vi "Read Digital Outputs Status.vi"(8 "error in (no error)":errorcluster, 11 "PXI6521 in":refnum<class "PXI6521.lvclass">) -> (0 "error out":errorcluster, 2 "Digital Outputs Status":bool[](array[boolean]), 3 "PXI6521 out":refnum<class "PXI6521.lvclass">)   [LabVIEW 2018, in "PXI6521.lvlib" / "PXI6521.lvclass"]
doc: "This VI reads the state of the Digital Outputs. The state is atores in the applicable class property."
uses:
  PXI6521.lvclass
  Custom Controls/DAQmx Lines Scope.ctl
  Custom Controls/DAQmx Digital Scope.ctl
  PXI6521.lvclass/PXI6521.ctl
  <vilib>/DAQmx/read.llb/DAQmx Read (Digital 1D Bool 1Chan 1Samp).vi
  <vilib>/DAQmx/create/channels.llb/DAQmx Create Channel (DO-Digital Output).vi
  <vilib>/DAQmx/miscellaneous.llb/DAQmx Fill In Error Info.vi
  PPLs/DigitalIO/Parent/DigitalIO.lvlibp/DigitalIO.lvclass
  C:/Projects/LabVIEW/PPLs/DigitalIO/Parent/DigitalIO.lvlibp/DigitalIO.lvclass
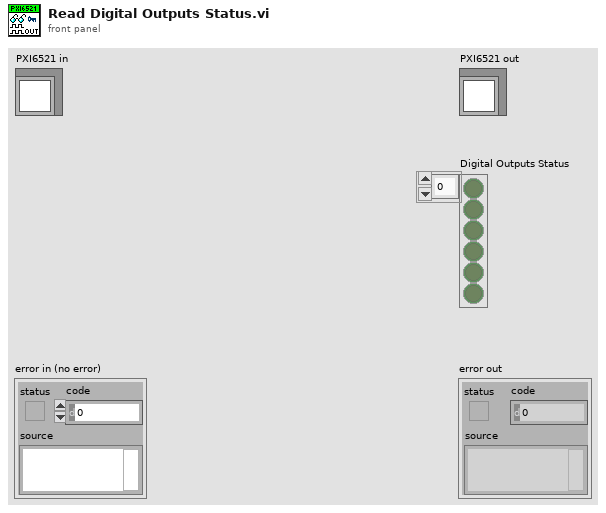
[diagram p1: front panel]
types:
  T1 = typedef "PXI6521.lvlib/PXI6521.lvclass/DAQmx Digital Scope.ctl" = enum16{"Input", "Output"}
  T2 = typedef "PXI6521.lvlib/PXI6521.lvclass/DAQmx Lines Scope.ctl" = enum16{"Full Range", "Custom Range", "Single"}
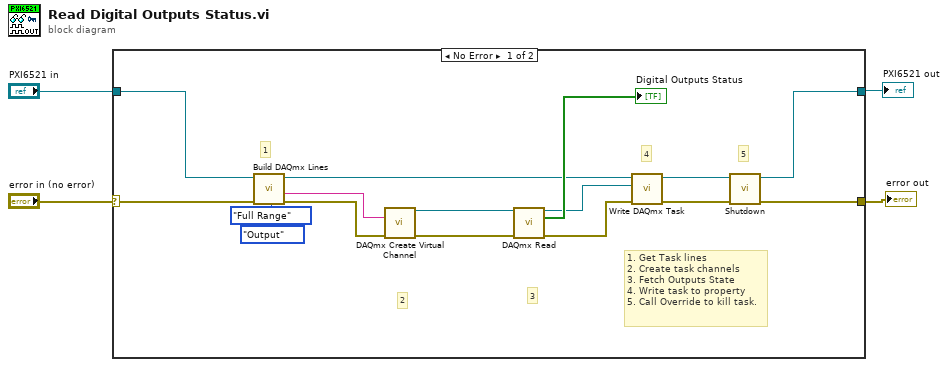
[diagram p0: block diagram]
diagram:
  n1 = case shown="No Error" "error in (no error)" {
    selector: "error in (no error)" -> [w13 w22]
    tunnel: [w6 w22] -> w3
    tunnel: [w5 w21] -> w1
    tunnel: "PXI6521 in" -> [w14 w21]
    frame No Error {
      # "1. Get Task lines\n2. Create task channels\n3. Fetch Outputs State\n4. Write task to property\n5. Call Override to kill task."
      # "5"
      # "4"
      # "3"
      # "2"
      # "1"
      n2 = call "Build DAQmx Lines.vi"("error in (no error)"=w13, "DAQmx Digital Scope"=DAQmx_Digital_Scope."Output", "DAQmx Lines Scope"=DAQmx_Lines_Scope."Full Range", "PXI6521 in"=w14) -> ("error out"=w12:errorcluster, "Full Line"=w18:string, "PXI6521 out"=w11:refnum<class "PXI6521.lvclass">)  [unwired: 5 in]
      n3 = call-poly <vilib>:"DAQmx Create Virtual Channel.vi"("lines"=w18, "error in"=w12) -> ("task out"=w17:refnum<k21>, "error out"=w16:errorcluster)  [unwired: 12 in]
      n4 = call-poly <vilib>:"DAQmx Read.vi"("task/channels in"=w17, "error in"=w16) -> ("task out"=w9:refnum<k21>, "data"=→"Digital Outputs Status":bool[], "error out"=w10:errorcluster)  [unwired: 11 in]
      n5 = call "Write DAQmx Task.vi"("error in (no error)"=w10, "DAQmx Task"=w9, "PXI6521 in"=w11) -> ("error out"=w7:errorcluster, "PXI6521 out"=w8:refnum<class "PXI6521.lvclass">)  [unwired: 7 in]
      n6 = call "Shutdown.vi"("error in (no error)"=w7, "DigitalIO in"=w8) -> ("error out"=w6:errorcluster, "DigitalIO out"=w5:refnum<class "PXI6521.lvclass">)  [unwired: 8 in]
    }
    frame Error {
    }
  }
  "error out" <- w3
  "PXI6521 out" <- w1
